vi "HFRR ADV v019 new software.vi"() -> ()   [LabVIEW 2025] (continued)
                n3037 = Concatenate Strings(w3752, "," ("string"), w3740, w3742, w3741, w3824, w3827, w3741, w3825, w3826, w3752) -> (w3750:string)
                n3038 = local read "Tested by"() -> (w3756:string)
                n3039 = local read "String 33"() -> (w3757:string)
                n3040 = Concatenate Strings("," ("string"), "                                                                             " ("string")) -> (w3745:string)
                n3041 = Concatenate Strings(w3747, w3743, w3750, w3743, w3753, w3782, w3743, w3745, w3757, w3756) -> (→"export":string)
                n3042 = String To Path(string=w3784) -> (path=w3791:path)
                n3043 = local read "export"() -> (w3786:string)
                n3044 = call <vilib>:"Write Characters To File.vi"("append to file? (new file:F)"=FALSE, "character string"=w3786, "file path (dialog if empty)"=w3791) -> ()  [unwired: 2 in, 1 out]
              }
            }
          }
          frame Enabled {
          }
        }
        n3045 = case shown="True" "OK Button 17" {
          frame False {
          }
          frame True {
            (unwired) 0  # existing file
            w4044 = "Choose a datalog file to open"  # prompt
            n3046 = local write "OK Button 17"(FALSE ("OK Button 17")) -> ()
            n3047 = local read "String"() -> (w4039:string)
            n3048 = String To Path(string=w4039) -> (path=w4040:path)
            n3049 = File Dialog(6:"*.duf" ("pattern"), 7:w4044, 11:w4040) -> (0:w4031:errorcluster, 3:w4050:path)  [unwired: 4 in, 2 out]
            n3050 = Unbundle(w4031) -> ()  [unwired: 3 out]
            n3051 = Open/Create/Replace File "Open File"(file path (use dialog)=w4050) -> (refnum out=w4042:refnum<file>)  [unwired: 5 in, 2 out]
            n3052 = Strip Path(path=w4050) -> (name=w4048:string)  [unwired: 1 out]
            n3053 = Path To String(path=w4050) -> (string=w4033:string)
            n3054 = while {
              tunnel: w4042 -> [w4054]
              i -> [w4051]
              stop <- w4052 continue-if-true
              (unwired) TRUE ("line mode (F)")
              n3055 = Read from Text File "Read File"(file (use dialog)=w4054) -> (text=w4053:string)  [unwired: 3 in, 3 out]
              n3056 = local write "Numeric 16"(w4051) -> ()
              n3057 = String Length(string=w4053) -> (length=w4056:i32)
              n3058 = Greater?(x=w4056, y=1) -> (0:w4052:bool)
            }
            n3059 = local write "String 29"(w4033) -> ()
            n3060 = Search and Replace String(input string=w4033, search string=".duf", replace string=".dgf" ("replace string (\"\")")) -> (result string=→"String Indicator 4":string)  [unwired: 5 in, 3 out]
            n3061 = Match Pattern(string=w4048, regular expression=".dwm") -> (before substring=w4032:string)  [unwired: 1 in, 3 out]
            "String Indicator" <- w4032
            n3062 = Match Pattern(string=w4033, regular expression=".dwm" ("substring (\"\")")) -> (before substring=w4034:string)  [unwired: 1 in, 3 out]
            "String Indicator 3" <- w4034
            n3063 = local write "TITTLE 2"(w4032) -> ()
            n3064 = String To Path(string=w4034) -> (path=w4041:path)
            "path" <- w4041
            n3065 = call <vilib>:"Read Characters From File.vi"("file path (dialog if empty)"=w4041, "start of read offset (chars.:0)"=60 ("start of read offset (chars.: 0)")) -> ("character string"=→"String Indicator 2":string)  [unwired: 4 in, 3 out]
          }
        }
        n3066 = call <vilib>:"Query Available Printers.vi"() -> ("system configured printers"=w3733:string[])  [unwired: 9 in, 2 out]
        "System Configured Printers 2" <- w3733
        n3067 = local read "OK Button 16"() -> (w3730:bool)
        n3068 = case shown="True" "OK Button 16" {
          frame False {
          }
          frame True {
            n3069 = stacked-sequence {
              frame #0 {
                n3070 = local read "Numeric 16"() -> (w4058:i32)
                n3071 = local write "Numeric 10"(w4058) -> ()
              }
              frame #1 {
                n3072 = local read "S.NO"() -> (→"s.NO":string)
                n3073 = local read "String 29"() -> (w4062:string)
                n3074 = String To Path(string=w4062) -> (path=w4061:path)
                n3075 = Open/Create/Replace File "Open File"(file path (use dialog)=w4061) -> (refnum out=w4063:refnum<file>)  [unwired: 5 in, 2 out]
                n3076 = for {
                  N: 16 -> [_]
                  tunnel: w4063 -> [w4070]
                  i -> [w4066]
                  (unwired) TRUE ("line mode (F)")
                  n3077 = Read from Text File "Read File"(file (use dialog)=w4070) -> (text=w4064:string)  [unwired: 3 in, 3 out]
                  n3078 = Match Pattern(string=w4064, regular expression="(") -> (after substring=w4069:string)  [unwired: 1 in, 3 out]
                  n3079 = Match Pattern(string=w4069, regular expression=")") -> (before substring=w4065:string)  [unwired: 1 in, 3 out]
                  n3080 = case shown="1" w4066 {
                    tunnel: w4065 -> [w4071 w4072 _ _ w4073 w4074 w4075 w4077 w4079 w4081 w4083 w4085 w4087 w4089 _]
                    tunnel: w4064 -> [_ _ _ _ _ _ _ _ _ _ _ _ _ _ _]
                    frame 0 {
                      "TITTLE" <- w4071
                    }
                    frame 1 {
                      "Sample ID" <- w4072
                    }
                    frame 2 {
                    }
                    frame 3 {
                    }
                    frame 4 {
                      "Test Date" <- w4073
                    }
                    frame 5 {
                      "Tested by" <- w4074
                    }
                    frame 6 {
                      n3081 = Fract/Exp String To Number(string=w4075) -> (number=→"Humidity before test 2":dbl)  [unwired: 3 in, 1 out]
                    }
                    frame 7 {
                      n3082 = Fract/Exp String To Number(string=w4077) -> (number=→"Temperature before test 2":dbl)  [unwired: 3 in, 1 out]
                    }
                    frame 8 {
                      n3083 = Fract/Exp String To Number(string=w4079) -> (number=→"Humidity after test 2":dbl)  [unwired: 3 in, 1 out]
                    }
                    frame 9 {
                      n3084 = Fract/Exp String To Number(string=w4081) -> (number=→"Temperature after test 2":dbl)  [unwired: 3 in, 1 out]
                    }
                    frame 10 {
                      n3085 = Fract/Exp String To Number(string=w4083) -> (number=→"MWSD 2":dbl)  [unwired: 3 in, 1 out]
                    }
                    frame 11 {
                      n3086 = Fract/Exp String To Number(string=w4085) -> (number=→"AVP 2":dbl)  [unwired: 3 in, 1 out]
                    }
                    frame 12 {
                      n3087 = Fract/Exp String To Number(string=w4087) -> (number=→"HCF 2":dbl)  [unwired: 3 in, 1 out]
                    }
                    frame 13 {
                      n3088 = Fract/Exp String To Number(string=w4089) -> (number=→"WS1.4 2":dbl)  [unwired: 3 in, 1 out]
                    }
                    frame 14, Default {
                    }
                  }
                }
              }
              frame #2 {
              }
            }
            n3089 = local write "OK Button 16"(FALSE ("OK Button 13")) -> ()
          }
        }
        n3090 = Index Array(array=w3733, index="Select Printer 3") -> (element=w3735:string)
        "Selected Printer" <- w3735
        n3091 = case shown="True" w3730 {
          frame False {
          }
          frame True {
            n3092 = flat-sequence {
              frame #0 {
              }
              frame #1 {
                n3093 = Wait (ms)(milliseconds to wait=u32 100) -> ()  [unwired: 1 out]
              }
              frame #2 {
                n3094 = local write "OK Button 16"(FALSE ("Print 3")) -> ()
              }
            }
          }
        }
        n3095 = case shown="True" "Print" {
          tunnel: w3735 -> [_ w4027]
          frame False {
          }
          frame True {
            (unwired) i16 6 ("width (-)")
            (unwired) "TESTED BY : "
            (unwired) "TESTED DATE :"
            (unwired) "SAMPLE ID : "
            (unwired) "SAMPLE DESIGN : "
            w3985 = "\r"
            w4002 = "\r"
            # "add image"
            n3096 = local read "Sample ID"() -> (w3975:string)
            n3097 = local read "Tested by"() -> (w3978:string)
            n3098 = local read "String 34"() -> (w3965:string)
            n3099 = local read "String 45"() -> (w3945:string)
            n3100 = local read "String 35"() -> (w3960:string)
            n3101 = local read "String 37"() -> (w3958:string)
            n3102 = local read "String 32"() -> (w3980:string)
            n3103 = local read "String 36"() -> (w3955:string)
            n3104 = local read "String 31"() -> (w3979:string)
            n3105 = local read "Test Date"() -> (w3976:string)
            n3106 = local read "String 33"() -> (w3981:string)
            n3107 = local read "String 38"() -> (w3951:string)
            n3108 = local read "String 39"() -> (w3948:string)
            n3109 = local write "Print"(FALSE ("Print FF")) -> ()
            n3110 = local read "S 39"() -> (w3963:string)
            n3111 = local read "S 38"() -> (w3970:string)
            n3112 = local read "Temperature before test 2"() -> (w4001:dbl)
            n3113 = local read "Temperature after test 2"() -> (w3991:dbl)
            n3114 = local read "Humidity before test 2"() -> (w4016:dbl)
            n3115 = local read "Humidity after test 2"() -> (w4000:dbl)
            n3116 = local read "MWSD 2"() -> (w4005:dbl)
            n3117 = local read "WS1.4 2"() -> (w3983:dbl)
            n3118 = Concatenate Strings("2)" ("string"), w3965) -> (w3966:string)
            n3119 = Concatenate Strings("3)" ("string"), w3963) -> (w3964:string)
            n3120 = Concatenate Strings("1)" ("string"), w3970) -> (w3969:string)
            n3121 = Concatenate Strings("4)" ("string"), w3960) -> (w3961:string)
            n3122 = Concatenate Strings("5)" ("string"), w3958) -> (w3957:string)
            n3123 = Concatenate Strings("6)" ("string"), w3955) -> (w3954:string)
            n3124 = Concatenate Strings("7)" ("string"), w3951) -> (w3952:string)
            n3125 = Concatenate Strings("8)" ("string"), w3948) -> (w3949:string)
            n3126 = local read "HCF 2"() -> (w3987:dbl)
            n3127 = local read "AVP 2"() -> (w4004:dbl)
            n3128 = local read "s.NO"() -> (w3946:string)
            n3129 = call <vilib>:"New Report.vi"("report type"=enum16{"Standard Report", "HTML"}."Standard Report") -> ("report out"=w4025:refnum<class "NI_report.lvclass">, "error out"=w4024:errorcluster)  [unwired: 13 in]
            n3130 = local read "TITTLE"() -> (w3977:string)
            n3131 = Concatenate Strings(w4002, w3945, w3946, w4002, w3980, w3975, w4002, w3979, w3976, w4002, w3981, w3978, w4002) -> (w3995:string)
            "test by" <- w3995
            n3132 = Number To Fractional String(number=w4001, width (-)=i16 6, precision (6)=i16 2) -> (F-format string=w3990:string)  [unwired: 1 in]
            n3133 = Number To Fractional String(number=w4000, width (-)=i16 6, precision (6)=i16 2) -> (F-format string=w4003:string)  [unwired: 1 in]
            n3134 = Number To Fractional String(number=w4016, width (-)=i16 6, precision (6)=i16 2) -> (F-format string=w4021:string)  [unwired: 1 in]
            n3135 = Number To Fractional String(number=w4005, width (-)=i16 6, precision (6)=i16 2) -> (F-format string=w4007:string)  [unwired: 1 in]
            n3136 = Number To Fractional String(number=w3991, width (-)=i16 6, precision (6)=i16 2) -> (F-format string=w3992:string)  [unwired: 1 in]
            n3137 = Number To Fractional String(number=w4004, width (-)=i16 6, precision (6)=i16 2) -> (F-format string=w4006:string)  [unwired: 1 in]
            n3138 = Number To Fractional String(number=w3987, width (-)=i16 6, precision (6)=i16 2) -> (F-format string=w3986:string)  [unwired: 1 in]
            n3139 = Number To Fractional String(number=w3983, precision (6)=i16 2) -> (F-format string=w3982:string)  [unwired: 2 in]
            n3140 = call-dynamic "Set Report Header Text.vi"("report in"=w4025, "center header text"=w3977, "error in (no error)"=w4024) -> ("report out"=w3996:refnum<class "NI_report.lvclass">, "error out"=w3997:errorcluster)  [unwired: 11 in]
            n3141 = Concatenate Strings(w3985, w3969, w4021, w3985, w3966, w3990, w3985, w3964, w4003, w3985, w3961, w3992, w3985, w3957, w4007, w3985, w3954, w4006, w3985, w3952, w3986, w3985, w3949, w3982) -> (w3973:string)
            "export 2" <- w3973
            n3142 = call-poly <vilib>:"Append Report Text.vi"("report in"=w3996, "text"=w3995, "error in (no error)"=w3997) -> ("report out"=w3999:refnum<class "NI_report.lvclass">, "error out"=w3998:errorcluster)  [unwired: 9 in, 2 out]
            n3143 = local read "test by"() -> (w3972:string)
            n3144 = local read "TITTLE"() -> (w3974:string)
            n3145 = call-poly <vilib>:"Append Report Text.vi"("report in"=w3999, "error in (no error)"=w3998) -> ("report out"=w4020:refnum<class "NI_report.lvclass">, "error out"=w4018:errorcluster)  [unwired: 10 in, 2 out]
            n3146 = Concatenate Strings(w3974, w3973, w3972) -> (→"output":string)
            n3147 = call-poly <vilib>:"Append Report Text.vi"("report in"=w4020, "text"=w3973, "error in (no error)"=w4018) -> ("report out"=w4019:refnum<class "NI_report.lvclass">, "error out"=w4017:errorcluster)  [unwired: 9 in, 2 out]
            n3148 = call-dynamic "Print Report.vi"("report in"=w4019, "printer name (default)"=w4027, "error in (no error)"=w4017) -> ("report out"=w4029:refnum<class "NI_report.lvclass">, "error out"=w4030:errorcluster)  [unwired: 11 in]
            n3149 = call-dynamic "Dispose Report.vi"("report in"=w4029, "error in (no error)"=w4030) -> ()  [unwired: 13 in, 1 out]
          }
        }
        n3150 = case shown="True" "Print 2" {
          frame False {
          }
          frame True {
            n3151 = flat-sequence {
              frame #0 {
                n3152 = local read "s.NO"() -> (→"s.NO 2":string)
                n3153 = Wait (ms)(milliseconds to wait=u32 20) -> ()  [unwired: 1 out]
                n3154 = local read "Sample ID  3"() -> (→"Sample ID  6":string)
                n3155 = local read "Sample ID  4"() -> (→"Sample ID  7":string)
                n3156 = local read "Sample ID"() -> (→"Sample ID  2":string)
                n3157 = local read "Tested by"() -> (→"Tested by 2":string)
                n3158 = local read "Test Date"() -> (→"Test Date 2":string)
                n3159 = local read "Humidity after test 3"() -> (→"Humidity after test 4":dbl)
                n3160 = local read "Ref A Test Date :"() -> (→"TITTLE 4":string)
                n3161 = local read "Temperature before test 3"() -> (w3852:dbl)
                n3162 = local read "Temperature before test 3"() -> (→"Temperature after test 5":dbl)
                n3163 = local read "Temperature after test 3"() -> (→"Temperature after test 4":dbl)
                n3164 = local read "Humidity before test 3"() -> (→"Humidity before test 4":dbl)
                n3165 = local write "Temperature before test 3"(w3852) -> ()
                n3166 = local read "image data"() -> (w3843:T16)
                n3167 = String To Path(string="C:\\LAB-IQ\\im\\Temp_resized.jpg") -> (path=w3844:path)
                "path 2" <- w3844
                n3168 = call <vilib>:"Write JPEG File.vi"("image data"=w3843, "path to JPEG file"=w3844) -> ()  [unwired: 8 in, 2 out]
                "Ref A Test Date :" <- "Ref A Test Date :"
                "Ref B Test Date :" <- "Ref B Test Date :"
                "Ref B Scar Value :" <- "Ref B Scar Value :"
                "Ref A Scar Value :" <- "Ref A Scar Value :"
              }
              frame #1 {
                (unwired) HTML_Report_Image_Alignment."MIDDLE" ("alignment (default)")
                w3880 = u16 0 items=["portrait", "landscape"] ("orientation (portrait)")
                (unwired) HTML_Report_Image_Alignment."ABSMIDDLE" ("alignment (default)")
                (unwired) "TESTED BY : "
                (unwired) "TESTED DATE :"
                (unwired) "SAMPLE ID : "
                (unwired) "SAMPLE DESIGN : "
                w3913 = "\r"
                # "add image"
                n3169 = Wait (ms)(milliseconds to wait=u32 20) -> ()  [unwired: 1 out]
                n3170 = local read "Sample ID  2"() -> (w3906:string)
                n3171 = local read "Wear Scar X"() -> (w3878:dbl)
                "Length ( microns ) 2" <- w3878
                n3172 = local read "Wear Scar Y"() -> (w3877:dbl)
                "Wear Scar Y ( microns ) :" <- w3877
                n3173 = local read "Test Date 2"() -> (w3907:string)
                n3174 = local read "Tested by 2"() -> (w3908:string)
                n3175 = local read "String 46"() -> (w3904:string)
                n3176 = local read "String 48"() -> (w3910:string)
                n3177 = local read "String 47"() -> (w3909:string)
                n3178 = local read "String 49"() -> (w3911:string)
                n3179 = local read "String 10"() -> (w3864:string)
                n3180 = local read "s.NO 2"() -> (w3905:string)
                n3181 = Add(x=w3878, y=w3877) -> (x+y=w3876:dbl)
                n3182 = call <vilib>:"New Report.vi"("report type"=enum16{"Standard Report", "HTML"}."HTML") -> ("report out"=w3884:refnum<class "NI_report.lvclass">, "error out"=w3882:errorcluster)  [unwired: 13 in]
                n3183 = Concatenate Strings(w3913, w3904, w3905, w3913, w3910, w3906, w3913, w3909, w3907, w3913, w3911, w3908, w3913) -> (→"test by 2":string)
                n3184 = Concatenate Strings("C:\\LAB-IQ\\Data\\" ("string"), w3864, ".jpg" ("string")) -> ()  [unwired: 1 out]
                n3185 = Divide(x=w3876, y=2.0) -> (x/y=→"Mean Wear ( microns) :":dbl)
                n3186 = call-dynamic "Set Report Orientation.vi"("report in"=w3884, "orientation (portrait)"=w3880, "error in (no error)"=w3882) -> ("report out"=w3883:refnum<class "NI_report.lvclass">, "error out"=w3881:errorcluster)  [unwired: 11 in]
                n3187 = for {
                  N: 5 -> [_]
                  tunnel: w3883 -> [w3934]
                  tunnel: [w3933] -> w3862
                  tunnel: w3881 -> [w3932]
                  tunnel: [w3931] -> w3861
                  n3188 = call-dynamic "Set Report Tab Width.vi"("report in"=w3934, "error in (no error)"=w3932) -> ("report out"=w3933:refnum<class "NI_report.lvclass">, "error out"=w3931:errorcluster)  [unwired: 12 in]
                }
                n3189 = local read "TITTLE"() -> (w3879:string)
                n3190 = call-dynamic "Set Report Header Text.vi"("report in"=w3862, "center header text"=w3879, "error in (no error)"=w3861) -> ("report out"=w3900:refnum<class "NI_report.lvclass">, "error out"=w3899:errorcluster)  [unwired: 11 in]
                n3191 = for {
                  N: 1 -> [_]
                  tunnel: [w3938] -> w3886
                  tunnel: [w3937] -> w3885
                  tunnel: w3900 -> [w3936]
                  tunnel: w3899 -> [w3935]
                  n3192 = call-dynamic "New Report Line.vi"("report in"=w3936, "error in (no error)"=w3935) -> ("report out"=w3938:refnum<class "NI_report.lvclass">, "error out"=w3937:errorcluster)  [unwired: 12 in]
                }
                n3193 = for {
                  N: 2 -> [_]
                  tunnel: [w3930] -> w3892
                  tunnel: [w3929] -> w3891
                  tunnel: w3886 -> [w3928]
                  tunnel: w3885 -> [w3927]
                  n3194 = call-dynamic "New Report Line.vi"("report in"=w3928, "error in (no error)"=w3927) -> ("report out"=w3930:refnum<class "NI_report.lvclass">, "error out"=w3929:errorcluster)  [unwired: 12 in]
                }
                n3195 = for {
                  N: 25 -> [_]
                  tunnel: w3892 -> [w3926]
                  tunnel: w3891 -> [w3924]
                  tunnel: [w3925] -> w3895
                  tunnel: [w3923] -> w3894
                  n3196 = call-dynamic "Set Report Tab Width.vi"("report in"=w3926, "error in (no error)"=w3924) -> ("report out"=w3925:refnum<class "NI_report.lvclass">, "error out"=w3923:errorcluster)  [unwired: 12 in]
                }
                n3197 = control-ref of="Tab Control 9"() -> (w3890:refnum<vi>)
                n3198 = call-dynamic "Append Control Image to Report.vi"("report in"=w3895, "alignment (default)"=HTML_Report_Image_Alignment."ABSMIDDLE", "ctrl reference"=w3890, "error in (no error)"=w3894) -> ("report out"=w3889:refnum<class "NI_report.lvclass">, "error out"=w3888:errorcluster)  [unwired: 8 in, 2 out]
                n3199 = for {
                  N: 3 -> [_]
                  tunnel: [w3922] -> w3873
                  tunnel: [w3921] -> w3872
                  tunnel: w3889 -> [w3920]
                  tunnel: w3888 -> [w3919]
                  n3200 = call-dynamic "New Report Line.vi"("report in"=w3920, "error in (no error)"=w3919) -> ("report out"=w3922:refnum<class "NI_report.lvclass">, "error out"=w3921:errorcluster)  [unwired: 12 in]
                }
                n3201 = for {
                  N: 100 -> [_]
                  tunnel: w3873 -> [w3918]
                  tunnel: w3872 -> [w3916]
                  tunnel: [w3917] -> w3869
                  tunnel: [w3915] -> w3867
                  n3202 = call-dynamic "Set Report Tab Width.vi"("report in"=w3918, "error in (no error)"=w3916) -> ("report out"=w3917:refnum<class "NI_report.lvclass">, "error out"=w3915:errorcluster)  [unwired: 12 in]
                }
                n3203 = String To Path(string="C:\\LAB-IQ\\im\\Temp_resized.jpg") -> (path=w3859:path)
                n3204 = call-poly <vilib>:"Append Image to Report.vi"("report in"=w3869, "path or URL of image"=w3859, "error in (no error)"=w3867) -> ("report out"=w3868:refnum<class "NI_report.lvclass">, "error out"=w3866:errorcluster)  [unwired: 9 in, 2 out]
                n3205 = call-poly <vilib>:"Open HTML Report in Browser.vi"("report in"=w3868, "error in (no error)"=w3866) -> ("report out"=w3903:refnum<class "NI_report.lvclass">, "error out"=w3902:errorcluster)  [unwired: 11 in, 1 out]
                n3206 = call-dynamic "Dispose Report.vi"("report in"=w3903, "error in (no error)"=w3902) -> ()  [unwired: 13 in, 1 out]
              }
              frame #2 {
              }
              frame #3 {
                n3207 = disable-structure shown="Disabled" {
                  frame Disabled {
                    n3208 = local read "String 10"() -> (w3943:string)
                    n3209 = Concatenate Strings("C:\\LAB-IQ-NXT\\Data\\" ("string"), w3943, ".jpg" ("string")) -> (w3941:string)
                    n3210 = String To Path(string=w3941) -> (path=w3940:path)
                    n3211 = Delete(path (use dialog)=w3940) -> ()  [unwired: 4 in, 3 out]
                  }
                  frame Enabled {
                  }
                }
                n3212 = local write "Print 2"(FALSE ("Print")) -> ()
              }
            }
          }
        }
      }
    }
    n3213 = property on="SetTemp" class="DigNum (strict)"("Disabled"=w1879) -> ()  [unwired: 2 in, 2 out]
    n3214 = Multiply(x=w1869, y=w1871) -> (x*y=w1870:dbl)
    n3215 = local read "MWSD"() -> (w1868:dbl)
    n3216 = Add(x=w1870, y=w1868) -> (x+y=→"WS1.4":dbl)
    n3217 = Wait (ms)(milliseconds to wait=u32 50) -> ()  [unwired: 1 out]
    n3218 = Wait (ms)(milliseconds to wait=u32 50) -> ()  [unwired: 1 out]
    n3219 = local read "Quit"() -> (w1867:bool)
  }
  n3220 = VISA Close(VISA resource name=w39, error in (no error)=w38) -> ()  [unwired: 1 out]
  n3221 = while {
    tunnel: [w4104] -> w48
    shift-right: [w4097] -> _
    shift-left: 0.0 -> [w4100]
    shift-right: [w4096] -> _
    shift-left: 0.0 -> [w4099]
    shift-right: [w4095] -> _
    shift-left: 400.0 ("vc_cmd") -> [w4098]
    stop <- w4104 stop-if-true
    # "PID LOGIC"
    n3222 = local read "RUN"() -> (w4102:bool)
    n3223 = local read "Auto Start Temp"() -> (w4091:bool)
    n3224 = local read "Auto Start Test"() -> (w4101:bool)
    n3225 = local read "START TEMP"() -> (w4093:bool)
    n3226 = And(x=w4091, y=w4101) -> (x .and. y?=w4092:bool)
    n3227 = Or(x=w4102, y=w4092) -> (x .or. y?=w4103:bool)
    n3228 = And(x=w4103, y=w4093) -> (x .and. y?=w4094:bool)
    n3229 = Wait (ms)(milliseconds to wait=u32 20) -> ()  [unwired: 1 out]
    n3230 = case shown="True" w4094 {
      tunnel: [400.0 ("out_vc_cmd") w4124] -> w4095
      tunnel: [w4107 w4126] -> w4096
      tunnel: [w4107 w4125] -> w4097
      tunnel: w4100 -> [_ w4115]
      tunnel: w4099 -> [_ w4114]
      tunnel: w4098 -> [_ w4113]
      frame False {
        w4107 = 0.0 ("error_out")
      }
      frame True {
        n3231 = local read "Set Strk"() -> (w4110:dbl)
        n3232 = local read "LVDT STROKE"() -> (w4108:dbl)
        n3233 = Add(x=w4110, y="Add up Stroke") -> (x+y=w4111:dbl)
        n3234 = formula code="// Zero-Hardcode Explicit Positional-Form PID Engine\n// Inputs: target_stroke, measured_stroke, dt, prev_error, integral_accumulator_in, prev_vc_cmd\n//         kp, ki, kd, max_step_change, max_amplitude, min_amplitude, startup_cmd\n// Outputs: vc_cmd, error_out, out_error, integral_accumulator_out, out_vc_cmd\n\n// 1. Calculate Tracking Error\nfloat current_error = target_stroke - measured_stroke;\nerror_out = current_error;\n\n// 2. Compute Proportional Term\nfloat p_term = kp * current_error;\n\n// 3. Compute Derivative Term\nfloat d_term = 0.0;\nif (dt > 0.0) {\n    d_term = kd * ((current_error - prev_error) / dt);\n}\n\n// 4. Update and Accumulate Integral Term\nfloat current_integral = integral_accumulator_in + (current_error * dt);\nfloat i_term = ki * current_integral;\n\n// 5. Calculate Ideal Target Command\nfloat ideal_command = startup_cmd + p_term + i_term + d_term;\n\n// 6. Anti-Windup Protection (Back-calculation method)\nif (ideal_command > max_amplitude) {\n    float excess = ideal_command - max_amplitude;\n    if (ki > 0.0) {\n        current_integral -= excess / ki;\n    }\n    ideal_command = max_amplitude;\n} else if (ideal_command < min_amplitude) {\n    float excess = ideal_command - min_amplitude;\n    if (ki > 0.0) {\n        current_integral -= excess / ki;\n    }\n    ideal_command = min_amplitude;\n}\n\n// 7. Apply Loop Rate Limiting (Protects voice coil from large voltage steps)\nfloat raw_adjustment = ideal_command - prev_vc_cmd;\n\nif (raw_adjustment > max_step_change) {\n    raw_adjustment = max_step_change;\n} else if (raw_adjustment < -max_step_change) {\n    raw_adjustment = -max_step_change;\n}\n\nfloat next_vc_cmd = prev_vc_cmd + raw_adjustment;\n\n// Final Output Safety Safeguard Clamping\nif (next_vc_cmd > max_amplitude) {\n    next_vc_cmd = max_amplitude;\n} else if (next_vc_cmd < min_amplitude) {\n    next_vc_cmd = min_amplitude;\n}\n\n// 8. Map to Shift Registers for memory persistence\nvc_cmd = next_vc_cmd;\nout_error = current_error;                     \nintegral_accumulator_out = current_integral;  \nout_vc_cmd = next_vc_cmd;"("target_stroke"=w4111, "measured_stroke"=w4108, "dt"="dt", "integral_accumulator_in"=w4114, "prev_error"=w4115, "prev_vc_cmd"=w4113, "kp"="kp", "ki"="ki", "kd"="kd", "max_step_change"="max_step_change", "max_amplitude"="max_amplitude", "min_amplitude"="min_amplitude", "startup_cmd"="startup_cmd") -> ("vc_cmd"=w4130:dbl, "out_error"=w4125:dbl, "integral_accumulator_out"=w4126:dbl, "out_vc_cmd"=w4124:dbl)  [unwired: 1 out]
        "output Vpp" <- w4130
        n3235 = Number To Fractional String(number=w4130, precision (6)=i16 1) -> (F-format string=w4128:string)  [unwired: 2 in]
        n3236 = Concatenate Strings("DAC;" ("string"), w4128) -> (w4112:string)
        n3237 = local write "Command"(w4112) -> ()
        "prev_error" <- w4115
        "integral_accumulator_in" <- w4114
        "prev_vc_cmd" <- w4113
      }
    }
    n3238 = local read "Quit"() -> (w4104:bool)
  }
  n3239 = Or(x=w44, y=w43) -> (x .or. y?=w45:bool)
  n3240 = Or(x=w41, y=w45) -> (x .or. y?=w50:bool)
  n3241 = control-ref of="new picture"() -> ()  [unwired: 1 out]
  n3242 = Or(x=w53, y=w50) -> (x .or. y?=w47:bool)
  n3243 = Or(x=w47, y=w48) -> (x .or. y?=w42:bool)
  n3244 = while {
    tunnel: [w4131] -> w52
    i -> [w4138]
    stop <- w4131 stop-if-true
    n3245 = local read "Quit"() -> (w4131:bool)
    n3246 = Equal To 0?(x=w4138) -> (x = 0?=w4136:bool)
    n3247 = call "Elapsed Time3"("Time Target (s)"=45.0, "Auto Reset"=TRUE) -> ("Time has Elapsed"=w4135:bool)  [unwired: 10 in, 7 out]
    n3248 = Wait (ms)(milliseconds to wait=u32 50) -> ()  [unwired: 1 out]
    n3249 = Or(x=w4135, y=w4136) -> (x .or. y?=w4137:bool)
    n3250 = case shown="True" w4137 {
      frame False {
      }
      frame True {
        n3251 = call <vilib>:"System Exec.vi"("run minimized? (F)"=TRUE, "error in (no error)"="error in (no error)", "command line"="powercfg.exe -change -monitor-timeout-ac 0") -> ("error out"=w4149:errorcluster)  [unwired: 5 in, 3 out]
        n3252 = call <vilib>:"System Exec.vi"("run minimized? (F)"=TRUE, "error in (no error)"=w4149, "command line"="powercfg.exe -change -disk-timeout-ac 0") -> ("error out"=w4148:errorcluster)  [unwired: 5 in, 3 out]
        n3253 = call <vilib>:"System Exec.vi"("run minimized? (F)"=TRUE, "error in (no error)"=w4148, "command line"="powercfg.exe -change -standby-timeout-ac 0") -> ("error out"=w4147:errorcluster)  [unwired: 5 in, 3 out]
        n3254 = call <vilib>:"System Exec.vi"("run minimized? (F)"=TRUE, "error in (no error)"=w4147, "command line"="powercfg.exe -change -hibernate-timeout-ac 0") -> ("error out"=w4146:errorcluster)  [unwired: 5 in, 3 out]
        n3255 = call <vilib>:"Simple Error Handler.vi"("error in (no error)"=w4146) -> ("error out"=w4152:errorcluster)  [unwired: 4 in, 4 out]
        n3256 = call <vilib>:"Clear Errors.vi"("error in (no error)"=w4152) -> ("error out"=→"error out":errorcluster)  [unwired: 5 in, 1 out]
      }
    }
  }
  n3257 = Compound Arithmetic op=OR(w55, w42, w52) -> (w54:bool)
  n3258 = flat-sequence {
    tunnel: w54 -> [_]
    tunnel: [w4154] -> w20
    tunnel: w20 -> [_]
    frame #0 {
      n3259 = call "CLOSE CONNECTION.vi"() -> ("error out"=w4154:errorcluster)  [unwired: 11 in]
    }
    frame #1 {
      n3260 = Quit LabVIEW(quit? (T)=TRUE) -> ()
      n3261 = local write "Quit"(FALSE ("EXIT")) -> ()
    }
  }
  n3262 = property on="Heater Button" class="Bool (strict)"("Visible"=TRUE) -> ()  [unwired: 2 in, 2 out]
  n3263 = disable-structure shown="Disabled" {
    disable-tunnel: _ -> [w4160 _]
    disable-tunnel: _ -> [w4157 _]
    disable-tunnel: _ -> [w4158 _]
    frame Disabled {
      n3264 = disable-structure shown="Disabled" {
        disable-tunnel: [w4167 _] -> w4159
        frame Disabled {
          n3265 = while {
            shift-right: [w4209] -> w4165
            shift-left: errorcluster {"status"=TRUE, "code"=0, "source"="Init"} ("error out") -> [w4174]
            shift-right: [w4208] -> w4164
            shift-left: _ -> [w4175]
            shift-right: [w4207] -> _
            shift-left: "" -> [w4206]
            tunnel: [w4168] -> w4167
            shift-right: ["Set Rh"] -> _
            shift-left: 0.0 ("Set Rh") -> [w4200]
            tunnel: [w4177] -> _
            i -> [w4177]
            stop <- w4168 stop-if-true
            n3266 = flat-sequence {
              tunnel: w4174 -> [w4212]
              tunnel: [w4212] -> w4173
              frame #0 {
                n3267 = Wait (ms)(milliseconds to wait=u32 200) -> ()  [unwired: 1 out]
              }
            }
            n3268 = local read "Com Port 3"() -> (w4176:refnum<visa-resource-name>)
            n3269 = local read "Humidity Str Rec"() -> (w4178:string)
            n3270 = Not Equal?(x="Set Rh", y=w4200) -> (x != y?=w4205:bool)
            n3271 = Number To Decimal String(number="Set Rh") -> (decimal integer string=w4203:string)  [unwired: 1 in]
            n3272 = Not Equal?(x=w4176, y=w4175) -> (x != y?=w4171:bool)
            n3273 = Concatenate Strings("#setPoint00" ("string"), w4203) -> (w4204:string)
            n3274 = case shown="False" w4205 {
              tunnel: w4204 -> [_ w4224]
              frame False {
                n3275 = local read "Humidity"() -> (w4221:bool)
                n3276 = case shown="True" w4221 {
                  frame False {
                    n3277 = local write "Humidity Str Send"("stop" ("Humidity Str Send")) -> ()
                  }
                  frame True {
                    n3278 = local write "Humidity Str Send"("start" ("Humidity Str Send")) -> ()
                  }
                }
              }
              frame True {
                n3279 = local write "Humidity Str Send"(w4224) -> ()
              }
            }
            n3280 = Or(x=w4171) -> (y=w4169:bool, x .or. y?=w4170:bool)
            n3281 = String Subset(string=w4178, offset (0)=7) -> (substring=w4193:string)  [unwired: 1 in]
            n3282 = Match Pattern(string=w4178, regular expression="?") -> (offset past match=w4196:i32)  [unwired: 1 in, 3 out]
            n3283 = Match Pattern(string=w4178, regular expression="v") -> (offset past match=w4199:i32)  [unwired: 1 in, 3 out]
            n3284 = case shown="True" w4170 {
              tunnel: w4173 -> [w4210 _]
              tunnel: [w4210 errorcluster {"status"=TRUE, "code"=0, "source"="Init"} ("error out")] -> w4172
              frame False {
              }
              frame True {
              }
            }
            n3285 = Equal?(x=w4196, y=-1) -> (x = y?=w4180:bool)
            n3286 = Match Pattern(string=w4193, regular expression="g") -> (after substring=w4194:string, offset past match=w4185:i32)  [unwired: 1 in, 2 out]
            n3287 = Match Pattern(string=w4193, regular expression="y") -> (after substring=w4192:string, offset past match=w4186:i32)  [unwired: 1 in, 2 out]
            n3288 = Greater?(x=w4186, y=w4185) -> (0:w4191:bool)
            n3289 = Greater Or Equal To 0?(x=w4186) -> (x >= 0?=w4183:bool)
            n3290 = Greater Or Equal To 0?(x=w4185) -> (x >= 0?=w4184:bool)
            n3291 = Or(x=w4183, y=w4184) -> (x .or. y?=w4182:bool)
            n3292 = Greater Or Equal To 0?(x=w4199) -> (x >= 0?=w4181:bool)
            n3293 = Select(t=w4192, s=w4191, f=w4194) -> (s? t:f=w4187:string)
            n3294 = case shown="Error" w4172 {
              selector: w4172 -> [w4237 w4283]
              tunnel: [w4235 w4276] -> w4209
              tunnel: w4175 -> [w4238 w4282]
              tunnel: [w4236 w4285] -> w4208
              tunnel: w4206 -> [w4225 w4284]
              tunnel: [w4232 w4284] -> w4207
              frame No Error {
                n3295 = call "Elapsed Time7"() -> ("Time has Elapsed"=w4231:bool)  [unwired: 12 in, 7 out]
                n3296 = Not Equal?(x="Humidity Str Send", y=w4225) -> (x != y?=w4227:bool)
                n3297 = Or(x=w4227, y=w4231) -> (x .or. y?=w4230:bool)
                n3298 = Select(t="Humidity Str Send", s=w4227, f="vals" ("regular expression")) -> (s? t:f=w4226:string)
                n3299 = Or(x=w4230, y="Send") -> (x .or. y?=w4234:bool)
                n3300 = case shown="True" w4234 {
                  tunnel: [w4241 w4246] -> w4235
                  tunnel: w4238 -> [w4240 w4254]
                  tunnel: w4237 -> [w4241 w4253]
                  tunnel: [w4240 w4247] -> w4236
                  tunnel: w4226 -> [_ w4252]
                  tunnel: [w4239 w4243] -> w4232
                  tunnel: "Humidity Str Send" -> [_ w4244]
                  tunnel: w4227 -> [_ w4245]
                  tunnel: w4225 -> [w4239 w4242]
                  frame False {
                  }
                  frame True {
                    n3301 = flat-sequence {
                      tunnel: w4254 -> [w4262]
                      tunnel: w4253 -> [w4261]
                      tunnel: w4252 -> [w4258]
                      tunnel: [w4260] -> w4251
                      tunnel: [w4259] -> w4250
                      tunnel: w4251 -> [w4265]
                      tunnel: w4250 -> [w4264]
                      tunnel: [w4265] -> w4249
                      tunnel: [w4264] -> w4248
                      tunnel: w4249 -> [w4272]
                      tunnel: w4248 -> [w4271]
                      tunnel: [w4270] -> w4247
                      tunnel: [w4269] -> w4246
                      frame #0 {
                        n3302 = local write "Ser Led"(TRUE ("Boolean 4")) -> ()
                        n3303 = Concatenate Strings(w4258, "\r") -> (w4257:string)
                        n3304 = VISA Write(VISA resource name=w4262, write buffer=w4257, error in (no error)=w4261) -> (VISA resource name out=w4260:refnum<visa-resource-name>, error out=w4259:errorcluster)  [unwired: 1 out]
                      }
                      frame #1 {
                        n3305 = Wait (ms)(milliseconds to wait="wait") -> ()  [unwired: 1 out]
                      }
                      frame #2 {
                        w4267 = FALSE ("Send")
                        n3306 = property class="Instr"(reference=w4272, error in=w4271) -> (reference out=w4273:refnum<visa-resource-name>, error out=w4274:errorcluster, "Serial Settings:Number of Bytes at Serial Port"=w4266:u32)
                        n3307 = local write "Send"(w4267) -> ()
                        n3308 = local write "Ser Led"(w4267) -> ()
                        n3309 = VISA Read(VISA resource name=w4273, byte count=w4266, error in (no error)=w4274) -> (VISA resource name out=w4270:refnum<visa-resource-name>, read buffer=→"Humidity Str Rec":string, error out=w4269:errorcluster)  [unwired: 1 out]
                      }
                    }
                    n3310 = Select(t=w4244, s=w4245, f=w4242) -> (s? t:f=w4243:string)
                  }
                }
              }
              frame Error {
                w4290 = u16 0 items=["None"=0, "XON/XOFF"=1, "RTS/CTS"=2, "DTR/DSR"=4] ("flow control")
                w4286 = u16 0 items=["None", "Odd", "Even", "Mark", "Space"] ("parity")
                w4289 = u16 10 items=["1.0"=10, "1.5"=15, "2.0"=20] ("stop bits")
                n3311 = VISA Close(VISA resource name=w4282, error in (no error)=w4283) -> (error out=w4281:errorcluster)
                n3312 = local write "humid"("" ("humid")) -> ()
                n3313 = local write "Humidity Str Rec"("" ("Humidity Str Rec")) -> ()
                n3314 = call <vilib>:"Clear Errors.vi"("error in (no error)"=w4281) -> ("error out"=w4280:errorcluster)  [unwired: 5 in, 1 out]
                n3315 = local read "Com Port 3"() -> (w4279:refnum<visa-resource-name>)
                n3316 = call-poly "VISA Configure Serial Port"("VISA resource name"=w4279, "timeout (10sec)"=u32 1000, "termination char\n(0xA = '\\n' = LF)"=u8 10 ("termination char\n(0xA = '\\n' = LF)"), "Enable Termination\nChar (T)"=FALSE ("Enable Termination Char (T)"), "data bits (8)"=u16 8 ("data bits"), "parity (0:none)"=w4286, "error in (no error)"=w4280, "stop bits (10: 1 bit)"=w4289, "flow control (0:none)"=w4290) -> ("VISA resource name out"=w4285:refnum<visa-resource-name>, "baud rate (9600)"=w4277:u32, "error out"=w4276:errorcluster)  [unwired: 4 in]
              }
            }
            n3317 = Compound Arithmetic op=AND(w4181, w4180, w4182) -> (w4179:bool)
            n3318 = case shown="True" w4179 {
              tunnel: w4178 -> [_ _]
              tunnel: w4187 -> [_ w4217]
              frame False {
              }
              frame True {
                w4215 = " " ("regular expression")
                n3319 = Match Pattern(string=w4217, regular expression=" ") -> (after substring=w4219:string)  [unwired: 1 in, 3 out]
                n3320 = Match Pattern(string=w4219, regular expression=w4215) -> (before substring=→"humid":string, after substring=w4216:string)  [unwired: 1 in, 2 out]
                n3321 = Match Pattern(string=w4216, regular expression=w4215) -> (before substring=→"temp_@Rh sensor":string)  [unwired: 1 in, 3 out]
              }
            }
            n3322 = local read "Quit"() -> (w4168:bool)
          }
          n3323 = VISA Close(VISA resource name=w4164, error in (no error)=w4165) -> (error out=w4161:errorcluster)
          n3324 = call <vilib>:"Clear Errors.vi"("error in (no error)"=w4161) -> ()  [unwired: 5 in, 2 out]
        }
        frame Enabled {
        }
      }
    }
    frame Enabled {
    }
  }
  n3325 = while {
    tunnel: [w4297] -> _
    i -> [w4297]
    stop <- w4293 stop-if-true
    # "Langauage selection"
    n3326 = Equal?(x="Lan flag", y=22.0) -> ()  [unwired: 1 out]
    n3327 = disable-structure shown="Disabled" {
      frame Disabled {
        n3328 = stacked-sequence {
          frame #0 {
            n3329 = case shown="\"Russian\"" "Language Selection" {
              tunnel: [0 1] -> w4299
              frame "English", Default {
              }
              frame "Russian" {
              }
            }
            n3330 = for {
              N: 130 -> [_]
              tunnel: "Table" -> [w4308]
              tunnel: w4299 -> [w4307]
              i -> [w4306]
              n3331 = Index Array(array=w4308, index (row)=w4306, index (col)=w4307) -> (element=w4305:string)
              n3332 = case shown="123" w4306 {
                tunnel: w4305 -> [w4309 w4310 _ w4311 w4312 w4313 w4314 w4315 w4316 w4317 w4318 w4319 w4320 w4321 w4322 w4323 w4324 w4325 w4326 w4327 w4328 w4329 w4330 w4331 w4332 w4333 w4334 w4335 w4336 _ _ w4337 w4338 w4339 w4340 w4341 w4342 w4351 w4358 w4365 w4372 w4376 w4379 w4382 w4384 w4386 w4387 w4388 w4389 w4390 w4391 w4392 w4393 w4394 w4395 w4396 w4397 w4398 w4399 w4400 w4401 w4402 w4403 w4404 w4405 w4406 w4407 w4408 w4409 w4410 w4411 w4412 w4413 w4414 w4415 w4416 w4417 w4418 w4419 w4420 w4421 w4422 w4423 w4424 w4425 w4426 w4427 w4428 w4429 w4430 w4431 w4432 w4433 w4434 w4435 w4436 w4437 w4438 w4439 w4440 w4441 w4442 w4443 w4444 w4445 _ w4446 w4447 w4448 w4449 w4450 w4451 w4452 w4453 w4454 w4455 w4456 w4457 w4458 _ w4459 w4460 w4461 w4462 w4463 w4464 _]
                frame 0 {
                  n3333 = local write "S"(w4309) -> ()
                }
                frame 1 {
                  n3334 = local write "S 2"(w4310) -> ()
                }
                frame 2 {
                }
                frame 3 {
                  n3335 = local write "S 4"(w4311) -> ()
                }
                frame 4 {
                  n3336 = property on="FILE" class="Str"("Caption.Text"=w4312) -> ()  [unwired: 2 in, 2 out]
                }
                frame 5 {
                  n3337 = property on="Fuel Discription :" class="Str"("Caption.Text"=w4313) -> ()  [unwired: 2 in, 2 out]
                }
                frame 6 {
                  n3338 = property on="Remarks :" class="Str"("Caption.Text"=w4314) -> ()  [unwired: 2 in, 2 out]
                }
                frame 7 {
                  n3339 = property on="Save & Continue" class="Bool (strict)"("Boolean Text.Text"=w4315) -> ()  [unwired: 2 in, 2 out]
                }
                frame 8 {
                }
                frame 9 {
                  n3340 = property on="Set Hz" class="DigNum (strict)"("Caption.Text"=w4317) -> ()  [unwired: 2 in, 2 out]
                }
                frame 10 {
                  "String 3" <- w4318
                }
                frame 11 {
                  n3341 = property on="NORMAL LOAD" class="DigNum (strict)"("Caption.Text"=w4319) -> ()  [unwired: 2 in, 2 out]
                }
                frame 12 {
                  "String 5" <- w4320
                }
                frame 13 {
                  n3342 = property on="Set Temp" class="DigNum (strict)"("Caption.Text"=w4321) -> ()  [unwired: 2 in, 2 out]
                }
                frame 14 {
                  n3343 = local write "S 15"(w4322) -> ()
                }
                frame 15 {
                  n3344 = property on="Set Rh" class="DigNum (strict)"("Caption.Text"=w4323) -> ()  [unwired: 2 in, 2 out]
                }
                frame 16 {
                  "String 13" <- w4324
                  "String 26" <- w4324
                }
                frame 17 {
                  n3345 = local write "S 18"(w4325) -> ()
                }
                frame 18 {
                  "String 17" <- w4326
                }
                frame 19 {
                  n3346 = property on="test time" class="DigNum (strict)"("Caption.Text"=w4327) -> ()  [unwired: 2 in, 2 out]
                }
                frame 20 {
                  "String 18" <- w4328
                  "String 22" <- w4328
                }
                frame 21 {
                  n3347 = property on="Elapsed time" class="DigNum (strict)"("Caption.Text"=w4329) -> ()  [unwired: 2 in, 2 out]
                }
                frame 22 {
                  n3348 = property on="Samplingtime 2" class="DigNum (strict)"("Caption.Text"=w4330) -> ()  [unwired: 2 in, 2 out]
                }
                frame 23 {
                  "String 21" <- w4331
                }
                frame 24 {
                  n3349 = property on="Countdown" class="DigNum (strict)"("Caption.Text"=w4332) -> ()  [unwired: 2 in, 2 out]
                }
                frame 25 {
                  n3350 = property on="Countdown 2" class="DigNum (strict)"("Caption.Text"=w4333) -> ()  [unwired: 2 in, 2 out]
                }
                frame 26 {
                  n3351 = property on="Engage" class="Bool (strict)"("Boolean Text.Text"=w4334) -> ()  [unwired: 2 in, 2 out]
                }
                frame 27 {
                  n3352 = property on="Boolean  4" class="Bool (strict)"("Boolean Text.Text"=w4335) -> ()  [unwired: 2 in, 2 out]
                }
                frame 28 {
                  n3353 = property on="Test \nStatus" class="Bool (strict)"("Boolean Text.Text"=w4336) -> ()  [unwired: 2 in, 2 out]
                }
                frame 29 {
                }
                frame 30 {
                }
                frame 31 {
                }
                frame 32 {
                  n3354 = property on="RSTCOF" class="Bool"("Boolean Text.Text"=w4338) -> ()  [unwired: 2 in, 2 out]
                  n3355 = property on="RST FF" class="Bool"("Boolean Text.Text"=w4338) -> ()  [unwired: 2 in, 2 out]
                  n3356 = property on="RST TEMP" class="Bool"("Boolean Text.Text"=w4338) -> ()  [unwired: 2 in, 2 out]
                  n3357 = property on="RSTV1 3" class="Bool"("Boolean Text.Text"=w4338) -> ()  [unwired: 2 in, 2 out]
                  n3358 = property on="rstv2" class="Bool"("Boolean Text.Text"=w4338) -> ()  [unwired: 2 in, 2 out]
                  n3359 = property on="RSTV1 2" class="Bool"("Boolean Text.Text"=w4338) -> ()  [unwired: 2 in, 2 out]
                  n3360 = property on="RST CP" class="Bool"("Boolean Text.Text"=w4338) -> ()  [unwired: 2 in, 2 out]
                }
                frame 33 {
                  "S 61" <- w4339
                }
                frame 34 {
                  "String 23" <- w4340
                }
                frame 35 {
                  n3361 = property on="Rh Before" class="DigNum (strict)"("Caption.Text"=w4341) -> ()  [unwired: 2 in, 2 out]
                }
                frame 36 {
                  n3362 = Match Pattern(string=w4342, regular expression=",") -> (before substring=→"bs":string, after substring=→"as":string)  [unwired: 1 in, 2 out]
                  n3363 = property on="Rh After" class="DigNum (strict)"("Caption.Text"=w4342) -> ()  [unwired: 2 in, 2 out]
                }
                frame 37 {
                  n3364 = Match Pattern(string=w4351, regular expression=",") -> (before substring=w4350:string, after substring=w4349:string)  [unwired: 1 in, 2 out]
                  "bs" <- w4350
                  "as" <- w4349
                  n3365 = Concatenate Strings(w4350, w4349) -> (w4346:string)
                  n3366 = property on="Humidity before test 2" class="DigNum (strict)"("Caption.Text"=w4346) -> ()  [unwired: 2 in, 2 out]
                  n3367 = property on="Humidity before test" class="DigNum (strict)"("Caption.Text"=w4346) -> ()  [unwired: 2 in, 2 out]
                  n3368 = Concatenate Strings(w4346, "=" ("string")) -> (w4347:string)
                  n3369 = local write "S 38"(w4347) -> ()
                }
                frame 38 {
                  n3370 = Match Pattern(string=w4358, regular expression=",") -> (before substring=w4357:string, after substring=w4356:string)  [unwired: 1 in, 2 out]
                  "bs" <- w4357
                  "as" <- w4356
                  n3371 = Concatenate Strings(w4357, w4356) -> (w4353:string)
                  n3372 = property on="Humidity after test 2" class="DigNum (strict)"("Caption.Text"=w4353) -> ()  [unwired: 2 in, 2 out]
                  n3373 = Concatenate Strings(w4353, "=" ("string")) -> (w4355:string)
                  n3374 = property on="Humidity after test" class="DigNum (strict)"("Caption.Text"=w4353) -> ()  [unwired: 2 in, 2 out]
                  n3375 = local write "S 39"(w4355) -> ()
                }
                frame 39 {
                  n3376 = Match Pattern(string=w4365, regular expression=",") -> (before substring=w4364:string, after substring=w4363:string)  [unwired: 1 in, 2 out]
                  "bs" <- w4364
                  "as" <- w4363
                  n3377 = Concatenate Strings(w4364, w4363) -> (w4360:string)
                  n3378 = property on="Temperature before test 2" class="DigNum (strict)"("Caption.Text"=w4360) -> ()  [unwired: 2 in, 2 out]
                  n3379 = property on="Temperature before test" class="DigNum (strict)"("Caption.Text"=w4360) -> ()  [unwired: 2 in, 2 out]
                  n3380 = Concatenate Strings(w4360, "=" ("string")) -> (→"String 34":string)
                }
                frame 40 {
                  n3381 = Match Pattern(string=w4372, regular expression=",") -> (before substring=w4371:string, after substring=w4370:string)  [unwired: 1 in, 2 out]
                  "bs" <- w4371
                  "as" <- w4370
                  n3382 = Concatenate Strings(w4371, w4370) -> (w4367:string)
                  n3383 = property on="Temperature after test 2" class="DigNum (strict)"("Caption.Text"=w4367) -> ()  [unwired: 2 in, 2 out]
                  n3384 = Concatenate Strings(w4367, "=" ("string")) -> (→"String 35":string)
                  n3385 = property on="Temperature after test" class="DigNum (strict)"("Caption.Text"=w4367) -> ()  [unwired: 2 in, 2 out]
                }
                frame 41 {
                  n3386 = property on="AVP" class="DigNum (strict)"("Caption.Text"=w4376) -> ()  [unwired: 2 in, 2 out]
                  n3387 = property on="AVP 2" class="DigNum (strict)"("Caption.Text"=w4376) -> ()  [unwired: 2 in, 2 out]
                  n3388 = Concatenate Strings(w4376, "=" ("string")) -> (→"String 36":string)
                }
                frame 42 {
                  n3389 = property on="MWSD" class="DigNum (strict)"("Caption.Text"=w4379) -> ()  [unwired: 2 in, 2 out]
                  n3390 = property on="MWSD 2" class="DigNum (strict)"("Caption.Text"=w4379) -> ()  [unwired: 2 in, 2 out]
                  n3391 = Concatenate Strings(w4379, "=" ("string")) -> (→"String 37":string)
                }
                frame 43 {
                  n3392 = property on="HCF 2" class="DigNum (strict)"("Caption.Text"=w4382) -> ()  [unwired: 2 in, 2 out]
                  n3393 = property on="HCF" class="DigNum (strict)"("Caption.Text"=w4382) -> ()  [unwired: 2 in, 2 out]
                  n3394 = Concatenate Strings(w4382, "=" ("string")) -> (→"String 38":string)
                }
                frame 44 {
                  n3395 = Concatenate Strings(w4384, "=" ("string")) -> (→"String 39":string)
                  n3396 = property on="WS1.4 2" class="DigNum (strict)"("Caption.Text"=w4384) -> ()  [unwired: 2 in, 2 out]
                  n3397 = property on="WS1.4" class="DigNum (strict)"("Caption.Text"=w4384) -> ()  [unwired: 2 in, 2 out]
                }
                frame 45 {
                  n3398 = property on="Save Results" class="Bool (strict)"("Boolean Text.Text"=w4386) -> ()  [unwired: 2 in, 2 out]
                }
                frame 46 {
                  n3399 = local write "S 47"(w4387) -> ()
                }
                frame 47 {
                  n3400 = local write "S 48"(w4388) -> ()
                }
                frame 48 {
                  n3401 = local write "S 49"(w4389) -> ()
                }
                frame 49 {
                  n3402 = local write "S 50"(w4390) -> ()
                }
                frame 50 {
                  n3403 = local write "S 51"(w4391) -> ()
                }
                frame 51 {
                  n3404 = local write "S 52"(w4392) -> ()
                }
                frame 52 {
                  n3405 = local write "S 53"(w4393) -> ()
                }
                frame 53 {
                  n3406 = local write "S 54"(w4394) -> ()
                }
                frame 54 {
                  n3407 = local write "S 55"(w4395) -> ()
                }
                frame 55 {
                  n3408 = local write "S 56"(w4396) -> ()
                }
                frame 56 {
                  n3409 = local write "S 57"(w4397) -> ()
                }
                frame 57 {
                  n3410 = local write "S 58"(w4398) -> ()
                }
                frame 58 {
                  n3411 = local write "S 59"(w4399) -> ()
                }
                frame 59 {
                  n3412 = local write "S 60"(w4400) -> ()
                }
                frame 60 {
                  n3413 = local write "S 62"(w4401) -> ()
                }
                frame 61 {
                  n3414 = local write "S 63"(w4402) -> ()
                }
                frame 62 {
                  n3415 = local write "S 64"(w4403) -> ()
                }
                frame 63 {
                  n3416 = local write "S 65"(w4404) -> ()
                }
                frame 64 {
                  n3417 = local write "S 66"(w4405) -> ()
                }
                frame 65 {
                  n3418 = local write "S 67"(w4406) -> ()
                }
                frame 66 {
                  n3419 = local write "S 68"(w4407) -> ()
                }
                frame 67 {
                  n3420 = local write "S 69"(w4408) -> ()
                }
                frame 68 {
                  n3421 = local write "S 70"(w4409) -> ()
                }
                frame 69 {
                  n3422 = local write "S 71"(w4410) -> ()
                }
                frame 70 {
                  n3423 = local write "S 72"(w4411) -> ()
                }
                frame 71 {
                  n3424 = local write "S 73"(w4412) -> ()
                }
                frame 72 {
                  n3425 = local write "S 74"(w4413) -> ()
                }
                frame 73 {
                  n3426 = local write "S 75"(w4414) -> ()
                }
                frame 74 {
                  n3427 = local write "S 76"(w4415) -> ()
                }
                frame 75 {
                  n3428 = local write "S 77"(w4416) -> ()
                }
                frame 76 {
                  n3429 = local write "S 78"(w4417) -> ()
                }
                frame 77 {
                  n3430 = local write "S 79"(w4418) -> ()
                }
                frame 79 {
                  n3431 = property on="Sample Temperature ( °C )" class="XYGraph (strict)"("Y Scale.Name Label.Text"=w4419) -> ()  [unwired: 2 in, 2 out]
                }
                frame 80 {
                  n3432 = local write "S 81"(w4420) -> ()
                  n3433 = property on="Humidity ( %RH )" class="XYGraph (strict)"("Y Scale.Name Label.Text"=w4420) -> ()  [unwired: 2 in, 2 out]
                }
                frame 78 {
                  n3434 = property on="Air Temperature  ( °C )" class="XYGraph (strict)"("X Scale.Name Label.Text"=w4421) -> ()  [unwired: 2 in, 2 out]
                  n3435 = property on="Humidity ( %RH )" class="XYGraph (strict)"("X Scale.Name Label.Text"=w4421) -> ()  [unwired: 2 in, 2 out]
                  n3436 = property on="Sample Temperature ( °C )" class="XYGraph (strict)"("X Scale.Name Label.Text"=w4421) -> ()  [unwired: 2 in, 2 out]
                  n3437 = property on="Coefficient Of Friction" class="XYGraph (strict)"("X Scale.Name Label.Text"=w4421) -> ()  [unwired: 2 in, 2 out]
                }
                frame 81 {
                  n3438 = property on="Air Temperature  ( °C )" class="XYGraph (strict)"("Y Scale.Name Label.Text"=w4422) -> ()  [unwired: 2 in, 2 out]
                }
                frame 82 {
                  n3439 = local write "S 84"(w4423) -> ()
                }
                frame 83 {
                  n3440 = local write "S 85"(w4424) -> ()
                }
                frame 84 {
                  n3441 = local write "S 86"(w4425) -> ()
                }
                frame 85 {
                  n3442 = local write "S 87"(w4426) -> ()
                }
                frame 86 {
                  n3443 = local write "S 88"(w4427) -> ()
                }
                frame 87 {
                }
                frame 88 {
                  n3444 = local write "S 90"(w4429) -> ()
                }
                frame 89 {
                  n3445 = local write "S 91"(w4430) -> ()
                }
                frame 90 {
                  n3446 = local write "S 92"(w4431) -> ()
                }
                frame 91 {
                  n3447 = local write "S 93"(w4432) -> ()
                }
                frame 92 {
                  n3448 = local write "S 94"(w4433) -> ()
                }
                frame 93 {
                  n3449 = local write "S 95"(w4434) -> ()
                }
                frame 94 {
                  n3450 = local write "S 96"(w4435) -> ()
                }
                frame 95 {
                  n3451 = local write "S 97"(w4436) -> ()
                }
                frame 96 {
                  n3452 = local write "S 98"(w4437) -> ()
                }
                frame 97 {
                  n3453 = local write "S 99"(w4438) -> ()
                }
                frame 98 {
                  n3454 = local write "S 100"(w4439) -> ()
                }
                frame 99 {
                  n3455 = local write "S 101"(w4440) -> ()
                }
                frame 100 {
                  n3456 = local write "S 102"(w4441) -> ()
                }
                frame 101 {
                  n3457 = local write "S 103"(w4442) -> ()
                }
                frame 102 {
                  n3458 = local write "S 104"(w4443) -> ()
                }
                frame 103 {
                  n3459 = local write "S 105"(w4444) -> ()
                }
                frame 104 {
                  n3460 = local write "S 106"(w4445) -> ()
                }
                frame 105 {
                }
                frame 106 {
                  n3461 = property on="OK Button 17" class="Bool (strict)"("Boolean Text.Text"=w4446) -> ()  [unwired: 2 in, 2 out]
                }
                frame 107 {
                  n3462 = property on="OK Button 16" class="Bool (strict)"("Boolean Text.Text"=w4447) -> ()  [unwired: 2 in, 2 out]
                }
                frame 108 {
                  n3463 = property on="TITTLE" class="Str"("Caption.Text"=w4448) -> ()  [unwired: 2 in, 2 out]
                }
                frame 109 {
                  "String 30" <- w4449
                }
                frame 110 {
                  n3464 = property on="Test Date" class="Str"("Caption.Text"=w4450) -> ()  [unwired: 2 in, 2 out]
                  "String 31" <- w4450
                }
                frame 111 {
                  n3465 = property on="Sample ID" class="Str"("Caption.Text"=w4451) -> ()  [unwired: 2 in, 2 out]
                  "String 32" <- w4451
                }
                frame 112 {
                  n3466 = property on="Tested by" class="Str"("Caption.Text"=w4452) -> ()  [unwired: 2 in, 2 out]
                  "String 33" <- w4452
                }
                frame 113 {
                  n3467 = property on="System Configured Printers 2" class="Arr (strict)"("Caption.Text"=w4453) -> ()  [unwired: 2 in, 2 out]
                }
                frame 114 {
                  n3468 = property on="Selected Printer" class="Str"("Caption.Text"=w4454) -> ()  [unwired: 2 in, 2 out]
                }
                frame 115 {
                  n3469 = property on="Select Printer 3" class="DigNum (strict)"("Caption.Text"=w4455) -> ()  [unwired: 2 in, 2 out]
                }
                frame 116 {
                  n3470 = property on="Print" class="Bool (strict)"("Boolean Text.Text"=w4456) -> ()  [unwired: 2 in, 2 out]
                }
                frame 117 {
                  "String 41" <- w4457
                }
                frame 118 {
                  n3471 = property on="tested by" class="Str"("Caption.Text"=w4458) -> ()  [unwired: 2 in, 2 out]
                }
                frame 119 {
                }
                frame 120 {
                  n3472 = property on="Export" class="Bool (strict)"("Boolean Text.Text"=w4459) -> ()  [unwired: 2 in, 2 out]
                }
                frame 121 {
                  n3473 = property on="TEMP INTERCEPT:" class="DigNum (strict)"("Caption.Text"=w4460) -> ()  [unwired: 2 in, 2 out]
                }
                frame 122 {
                  n3474 = property on="AIR TEMP INTERCEPT:" class="DigNum (strict)"("Caption.Text"=w4461) -> ()  [unwired: 2 in, 2 out]
                }
                frame 123 {
                  n3475 = property on="Select File Type" class="Enum (strict)"("Caption.Text"=w4462) -> ()  [unwired: 2 in, 2 out]
                }
                frame 124 {
                  n3476 = property on="s.NO" class="Str"("Caption.Text"=w4463) -> ()  [unwired: 2 in, 2 out]
                  "String 45" <- w4463
                }
